vi "Nearest_neighbors.vi"(9 "n neighbors":i32, 10 "Membank":T1, 11 "Features":sgl[][](array[numeric])) -> (0 "locations":i32[][](array[numeric]), 1 "patch scores":sgl[][](array[numeric]), 2 "locations":i32[](array[numeric]), 3 "patch scores":sgl[](array[numeric]), 5 "exec time":dbl)   [LabVIEW 2020]
uses:
  API/Controls/MemBank_and_Norm_Variants.ctl
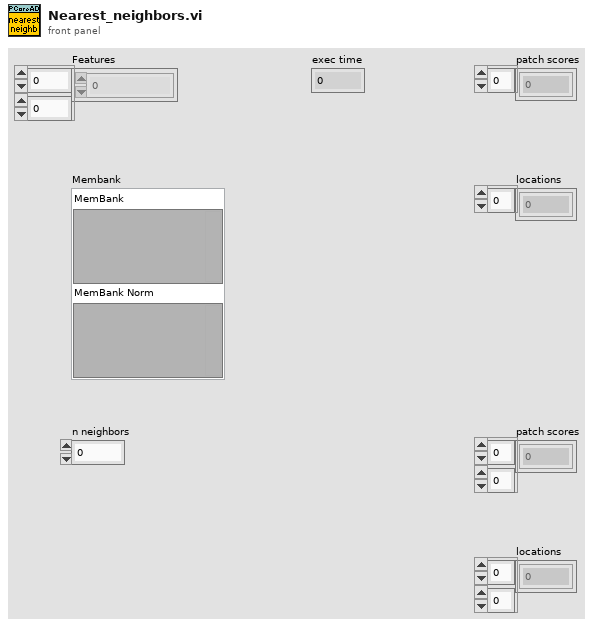
[diagram p1: front panel]
types:
  T1 = typedef "MemBank_and_Norm_Variants.ctl" = cluster{"MemBank":variant, "MemBank Norm":variant}
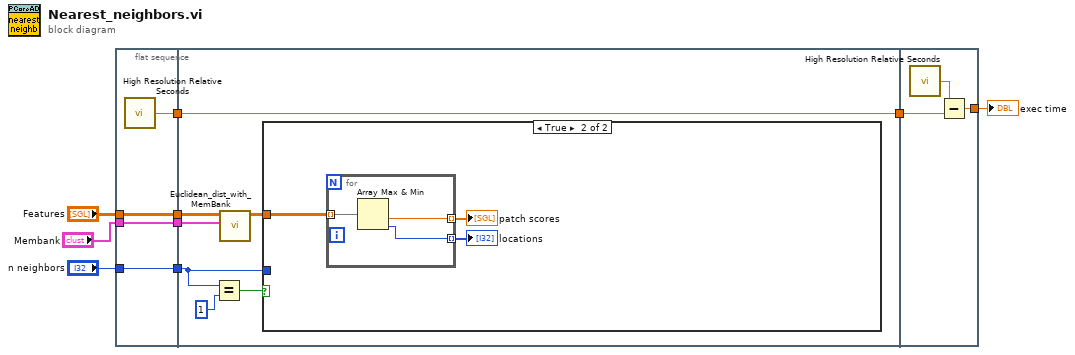
[diagram p0: block diagram]
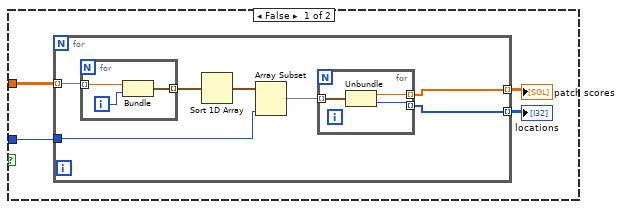
[diagram p2: hidden frame]
diagram:
  n1 = flat-sequence {
    tunnel: "n neighbors" -> [w12]
    tunnel: "Features" -> [w13]
    tunnel: [w13] -> w7
    tunnel: [w12] -> w6
    tunnel: [w11] -> w4
    tunnel: "Membank" -> [w10]
    tunnel: [w10] -> w2
    tunnel: w7 -> [w15]
    tunnel: w6 -> [w18]
    tunnel: [w17] -> w5
    tunnel: w4 -> [w17]
    tunnel: w2 -> [w16]
    tunnel: w5 -> [w45]
    tunnel: [w44] -> w3
    frame #0 {
      n2 = call <vilib>:"High Resolution Relative Seconds.vi"() -> ("relative seconds"=w11:dbl)
    }
    frame #1 {
      n3 = Equal?(x=w18, y=1) -> (x = y?=w19:bool)
      n4 = call "Euclidean_dist_with_MemBank.vi"("Membank"=w16, "x"=w15) -> ("distances"=w14:sgl[][])  [unwired: 7 in, 2 out]
      n5 = case shown="True" w19 {
        tunnel: w14 -> [w23 w40]
        tunnel: w18 -> [w24 _]
        frame False {
          n6 = for {
            tunnel: w23 -> [w31] mode=indexing
            tunnel: w24 -> [w28]
            tunnel: [w26] -> w22 mode=indexing
            tunnel: [w25] -> w21 mode=indexing
            n7 = for {
              tunnel: [w37] -> w30 mode=indexing
              tunnel: w31 -> [w36] mode=indexing
              i -> [w35]
              n8 = Bundle("Numeric"=w36, w35) -> (w37:cluster{"Numeric":sgl, i32})  [unwired: 1 in]
            }
            n9 = Sort 1D Array(array=w30) -> (sorted array=w29:cluster{"Numeric":sgl, i32}[])
            n10 = Array Subset(array=w29, length=w28) -> (w27:cluster{"Numeric":sgl, i32}[])  [unwired: 1 in]
            n11 = for {
              tunnel: w27 -> [w32] mode=indexing
              tunnel: [w34] -> w25 mode=indexing
              tunnel: [w33] -> w26 mode=indexing
              n12 = Unbundle(w32) -> ("Numeric"=w34:sgl, w33:i32)
            }
          }
          "locations" <- w22
          "patch scores" <- w21
        }
        frame True {
          n13 = for {
            tunnel: w40 -> [w43] mode=indexing
            tunnel: [w42] -> w38 mode=indexing
            tunnel: [w41] -> w39 mode=indexing
            n14 = Array Max & Min(array=w43) -> (min value=w42:sgl, min index (indices)=w41:i32)  [unwired: 2 out]
          }
          "patch scores" <- w38
          "locations" <- w39
        }
      }
    }
    frame #2 {
      n15 = call <vilib>:"High Resolution Relative Seconds.vi"() -> ("relative seconds"=w46:dbl)
      n16 = Subtract(x=w46, y=w45) -> (x-y=w44:dbl)
    }
  }
  "exec time" <- w3
